vi "WS104x_NI_6501_Relay_Control.vi"(0 "1P8_EN":bool=TRUE, 1 "RLY_2_SW_PIC":bool, 2 "RF_SW_CNT1":bool, 5 "VCO_CNT1":bool, 7 "RLY_1_SW_PIC":bool, 9 "RF_SW_CNT2":bool, 11 "error in":errorcluster, 12 "DIG_GND":bool) -> (15 "error out":errorcluster)   [LabVIEW 2012]
doc: "I. Description:\nThis example demonstrates how to write values to a digital output channel.\n\nII. Instructions for Running:\n1. Select the digital lines on the DAQ device to be written.\n2. Select a value to write.\nNote: The array control is sized for 8 lines, if using a different amount of lines, change the number of elements in the array to equal the number of lines chosen.\n\nIII. Block Diagram Steps:\n1. Create a Digital Output channel. Use one channel for all lines. You can alternatively use one channel for each line, but then use a different polymorphic version of the DAQmx Write VI.\n2. Call the Start VI to start the task.\n3. Write the digital Boolean array data in a loop until the user hits the stop button or an error occurs. This write VI writes a single sample of digital data on demand, so no timeout is necessary.\n4. Call the Clear Task VI to clear the Task.\n5. Use the popup dialog box to display an error or warning if any.\n\nIV. I/O Connections Overview:\nMake sure your signal output terminals match the Lines I/O Control. In this case wire the item to receive the signal to the first eight digital lines on your DAQ Device."
uses:
  <vilib>/DAQmx/create/channels.llb/DAQmx Create Channel (DO-Digital Output).vi
  <vilib>/DAQmx/write.llb/DAQmx Write (Digital Bool 1Line 1Point).vi
panel:
  in  "Lines 7":tag="Dev1/port0/line6" caption="Lines"
  in  "Lines 6":tag="Dev1/port0/line5" caption="Lines"
  in  "Lines 5":tag="Dev1/port0/line4" caption="Lines"
  in  "Lines 4":tag="Dev1/port0/line3" caption="Lines"
  in  "Lines 3":tag="Dev1/port0/line2" caption="Lines"
  in  "Lines 2":tag="Dev1/port0/line1" caption="Lines"
  in  "Lines":tag="Dev1/port0/line0"
  # "For instructions, select Help>>Show Context Help"
  # "Channel Parameters"
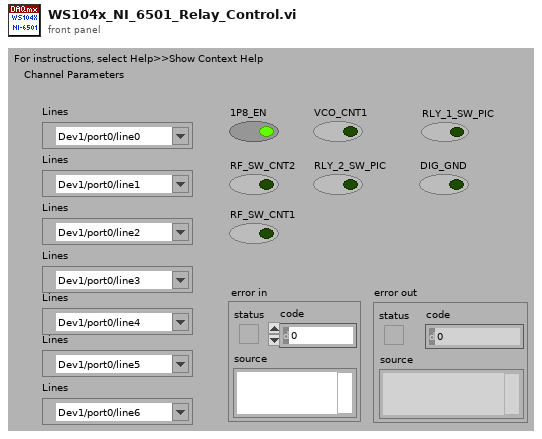
[diagram p1: front panel]
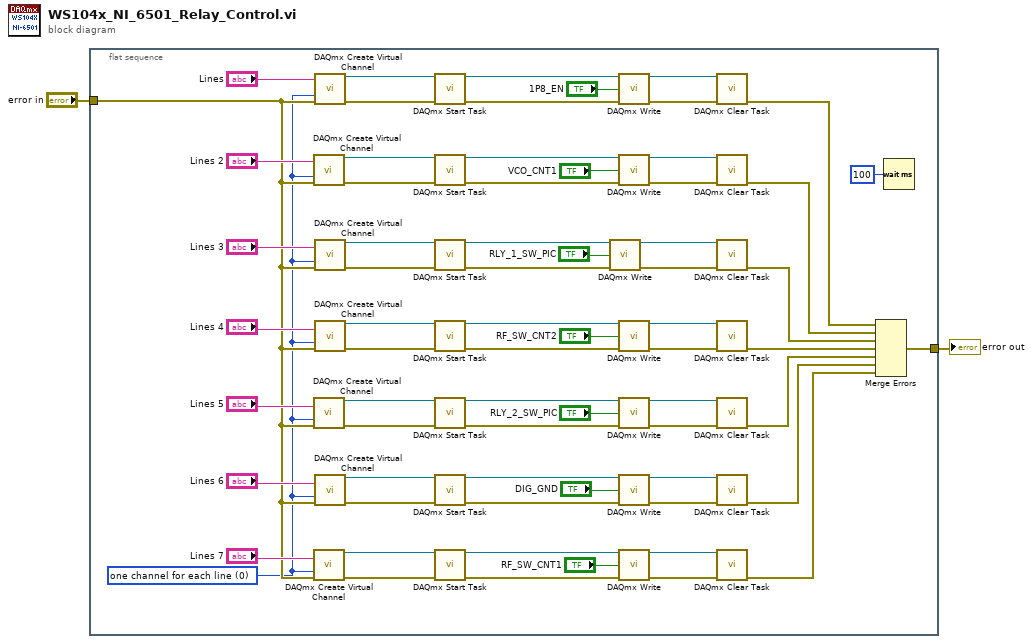
[diagram p0: block diagram]
diagram:
  n1 = flat-sequence {
    tunnel: "error in" -> [w13]
    tunnel: [w5] -> w1
    frame #0 {
      w3 = 0 items=["one channel for each line", "one channel for all lines"] ("line grouping")
      n2 = call-poly <vilib>:"DAQmx Create Virtual Channel.vi"("lines"="Lines 2", "line grouping"=w3, "error in"=w13) -> ("task out"=w58:refnum<k21>, "error out"=w59:errorcluster)  [unwired: 11 in]
      n3 = call-poly <vilib>:"DAQmx Create Virtual Channel.vi"("lines"="Lines 5", "line grouping"=w3, "error in"=w13) -> ("task out"=w33:refnum<k21>, "error out"=w32:errorcluster)  [unwired: 11 in]
      n4 = call-poly <vilib>:"DAQmx Create Virtual Channel.vi"("lines"="Lines 7", "line grouping"=w3, "error in"=w13) -> ("task out"=w17:refnum<k21>, "error out"=w16:errorcluster)  [unwired: 11 in]
      n5 = call-poly <vilib>:"DAQmx Create Virtual Channel.vi"("lines"="Lines", "line grouping"=w3, "error in"=w13) -> ("task out"=w65:refnum<k21>, "error out"=w64:errorcluster)  [unwired: 11 in]
      n6 = call-poly <vilib>:"DAQmx Create Virtual Channel.vi"("lines"="Lines 3", "line grouping"=w3, "error in"=w13) -> ("task out"=w49:refnum<k21>, "error out"=w48:errorcluster)  [unwired: 11 in]
      n7 = call-poly <vilib>:"DAQmx Create Virtual Channel.vi"("lines"="Lines 4", "line grouping"=w3, "error in"=w13) -> ("task out"=w42:refnum<k21>, "error out"=w43:errorcluster)  [unwired: 11 in]
      n8 = call-poly <vilib>:"DAQmx Create Virtual Channel.vi"("lines"="Lines 6", "line grouping"=w3, "error in"=w13) -> ("task out"=w27:refnum<k21>, "error out"=w28:errorcluster)  [unwired: 11 in]
      n9 = call <vilib>:"DAQmx Start Task.vi"("task/channels in"=w65, "error in"=w64) -> ("task out"=w67:refnum<k21>, "error out"=w69:errorcluster)  [unwired: 12 in]
      n10 = call <vilib>:"DAQmx Start Task.vi"("task/channels in"=w58, "error in"=w59) -> ("task out"=w56:refnum<k21>, "error out"=w54:errorcluster)  [unwired: 12 in]
      n11 = call <vilib>:"DAQmx Start Task.vi"("task/channels in"=w49, "error in"=w48) -> ("task out"=w51:refnum<k21>, "error out"=w53:errorcluster)  [unwired: 12 in]
      n12 = call <vilib>:"DAQmx Start Task.vi"("task/channels in"=w42, "error in"=w43) -> ("task out"=w40:refnum<k21>, "error out"=w38:errorcluster)  [unwired: 12 in]
      n13 = call <vilib>:"DAQmx Start Task.vi"("task/channels in"=w33, "error in"=w32) -> ("task out"=w35:refnum<k21>, "error out"=w37:errorcluster)  [unwired: 12 in]
      n14 = call <vilib>:"DAQmx Start Task.vi"("task/channels in"=w27, "error in"=w28) -> ("task out"=w25:refnum<k21>, "error out"=w23:errorcluster)  [unwired: 12 in]
      n15 = call <vilib>:"DAQmx Start Task.vi"("task/channels in"=w17, "error in"=w16) -> ("task out"=w19:refnum<k21>, "error out"=w21:errorcluster)  [unwired: 12 in]
      n16 = call-poly <vilib>:"DAQmx Write.vi"("task/channels in"=w51, "data"="RLY_1_SW_PIC", "error in"=w53) -> ("task out"=w50:refnum<k21>, "error out"=w52:errorcluster)  [unwired: 10 in, 1 out]
      n17 = call-poly <vilib>:"DAQmx Write.vi"("task/channels in"=w67, "data"="1P8_EN", "error in"=w69) -> ("task out"=w66:refnum<k21>, "error out"=w68:errorcluster)  [unwired: 10 in, 1 out]
      n18 = call-poly <vilib>:"DAQmx Write.vi"("task/channels in"=w56, "data"="VCO_CNT1", "error in"=w54) -> ("task out"=w57:refnum<k21>, "error out"=w55:errorcluster)  [unwired: 10 in, 1 out]
      n19 = call-poly <vilib>:"DAQmx Write.vi"("task/channels in"=w40, "data"="RF_SW_CNT2", "error in"=w38) -> ("task out"=w41:refnum<k21>, "error out"=w39:errorcluster)  [unwired: 10 in, 1 out]
      n20 = call-poly <vilib>:"DAQmx Write.vi"("task/channels in"=w35, "data"="RLY_2_SW_PIC", "error in"=w37) -> ("task out"=w34:refnum<k21>, "error out"=w36:errorcluster)  [unwired: 10 in, 1 out]
      n21 = call-poly <vilib>:"DAQmx Write.vi"("task/channels in"=w25, "data"="DIG_GND", "error in"=w23) -> ("task out"=w26:refnum<k21>, "error out"=w24:errorcluster)  [unwired: 10 in, 1 out]
      n22 = call-poly <vilib>:"DAQmx Write.vi"("task/channels in"=w19, "data"="RF_SW_CNT1", "error in"=w21) -> ("task out"=w18:refnum<k21>, "error out"=w20:errorcluster)  [unwired: 10 in, 1 out]
      n23 = call <vilib>:"DAQmx Clear Task.vi"("task in"=w66, "error in"=w68) -> ("error out"=w12:errorcluster)  [unwired: 13 in]
      n24 = call <vilib>:"DAQmx Clear Task.vi"("task in"=w57, "error in"=w55) -> ("error out"=w11:errorcluster)  [unwired: 13 in]
      n25 = call <vilib>:"DAQmx Clear Task.vi"("task in"=w50, "error in"=w52) -> ("error out"=w10:errorcluster)  [unwired: 13 in]
      n26 = call <vilib>:"DAQmx Clear Task.vi"("task in"=w41, "error in"=w39) -> ("error out"=w9:errorcluster)  [unwired: 13 in]
      n27 = call <vilib>:"DAQmx Clear Task.vi"("task in"=w34, "error in"=w36) -> ("error out"=w8:errorcluster)  [unwired: 13 in]
      n28 = call <vilib>:"DAQmx Clear Task.vi"("task in"=w26, "error in"=w24) -> ("error out"=w7:errorcluster)  [unwired: 13 in]
      n29 = call <vilib>:"DAQmx Clear Task.vi"("task in"=w18, "error in"=w20) -> ("error out"=w6:errorcluster)  [unwired: 13 in]
      n30 = Merge Errors(w12, w11, w10, w9, w8, w7, w6) -> (w5:errorcluster)
      n31 = Wait (ms)(milliseconds to wait=u32 100) -> ()  [unwired: 1 out]
    }
  }
  "error out" <- w1
